vi "PH_gentec_M-Link.set wanted Settings to GUI.vi"(0 "i ref in":refnum<vi>, 5 "error in":errorcluster) -> (14 "i ref out":refnum<vi>, 19 "error out":errorcluster)   [LabVIEW 2014, in "PH_gentec_M-Link.lvlib"]
doc: "This VI indicates the wanted Settings at the GUI element."
uses:
  PH_gentec_M-Link.lvlib
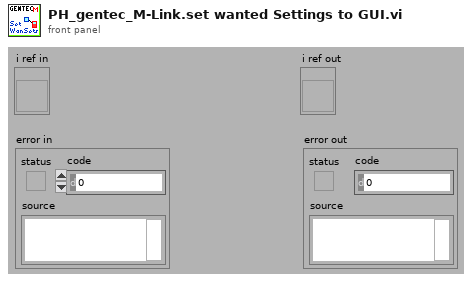
[diagram p1: front panel]
types:
  T1 = typedef "PH_gentec_M-Link.lvlib/PH_gentec_M-Link.i attribute.ctl" = cluster{"GUI References":cluster{"Wanted Head Settings":refnum<vi>, "Current Head Settings":refnum<vi>, "Set Auto Range":refnum<vi>, "Trigger Polarity":refnum<vi>, "Trigger Source":refnum<vi>, "Waveform Averages":refnum<vi>, "Continuous":refnum<vi>, "get one Value":refnum<vi>}, "Wanted Head Settings":T2, "Current Head Settings":T2}
  T2 = typedef "PH_gentec_M-Link.lvlib/PH_gentec_M-Link.Head Settings.ctl" = cluster{"Measurement Mode":T3, "Enable Anticipation":bool, "Set Auto Range":bool, "Block Signal":bool, "Set Head Attenuator":bool, "Enable SSE":bool, "Trigger Polarity":T4, "Trigger Source":T5, "Waveform Averages":T6, "Set Zero":i32, "Current":i32, "Start Data Flow":bool}
  T3 = typedef "gentec-M-Link - Driver.lvlib/gentec-M-Link.Measurement Mode.ctl" = u16
  T4 = typedef "gentec-M-Link - Driver.lvlib/gentec-M-Link.Trigger Polarity.ctl" = u16
  T5 = typedef "gentec-M-Link - Driver.lvlib/gentec-M-Link.Trigger Source.ctl" = u16
  T6 = typedef "gentec-M-Link - Driver.lvlib/gentec-M-Link.Waveform Averages.ctl" = u16
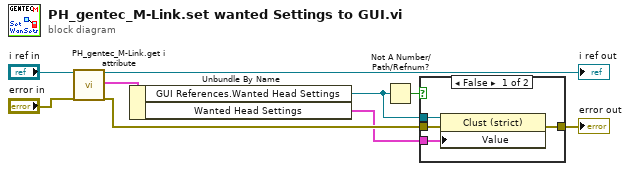
[diagram p0: block diagram]
diagram:
  n1 = call "PH_gentec_M-Link.get i attribute.vi"("i ref in"="i ref in", "error in (no error)"="error in") -> ("i ref out"=→"i ref out":refnum<vi>, "i attribute"=w8:T1, "error out"=w4:errorcluster)  [unwired: 15 in]
  n2 = Unbundle By Name(w8) -> ("GUI References.Wanted Head Settings"=w1:refnum<vi>, "Wanted Head Settings"=w3:T2)
  n3 = Not A Number/Path/Refnum?(number/path/refnum=w1) -> (NaN/Path/Refnum?=w2:bool)
  n4 = case shown="False" w2 {
    tunnel: [w13 w14] -> w9
    tunnel: w1 -> [w12 _]
    tunnel: w4 -> [w11 w14]
    tunnel: w3 -> [w10 _]
    frame False {
      n5 = property class="Clust (strict)"(reference=w12, error in=w11, "Value"=w10) -> (error out=w13:errorcluster)  [unwired: 1 out]
    }
    frame True {
    }
  }
  "error out" <- w9
